vi "Read Binary Config.vi"(4 "Class Name is Included":bool, 6 "byte order (0:big-endian, network order)":T1(ring), 8 "error in (no error)":errorcluster, 10 "Binary":string, 11 "AbsComp_One Term_STR in":refnum<class "AbsComp_One Term_STR.lvclass">) -> (0 "error out":errorcluster, 2 "Remaining":string, 3 "AbsComp_One Term_STR out":refnum<class "AbsComp_One Term_STR.lvclass">)   [LabVIEW 2021, in "AbsComp_One Term_STR.lvclass"]
uses:
  AbsComp_One Term_STR.lvclass
  Abs_Types/Boolean/Abs_Boolean.lvclass
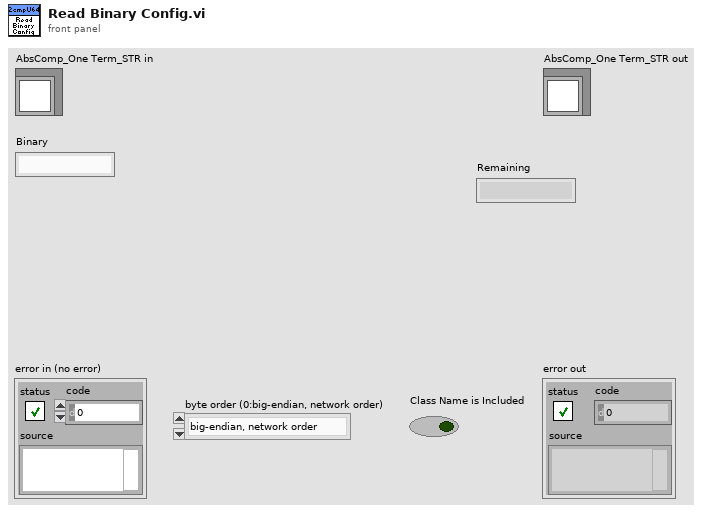
[diagram p1: front panel]
types:
  T1 = enum16{"big-endian, network order", "native, host order", "little-endian"}
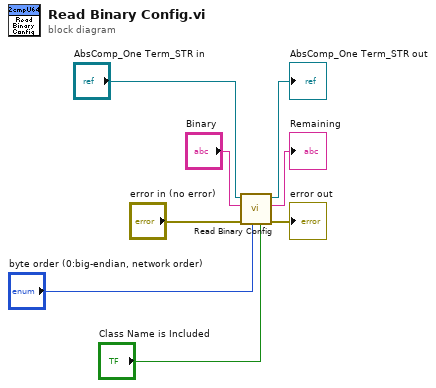
[diagram p0: block diagram]
diagram:
  n1 = call-parent "Read Binary Config.vi"("Class Name is Included"="Class Name is Included", "byte order (0:big-endian, network order)"="byte order (0:big-endian, network order)", "error in (no error)"="error in (no error)", "Binary"="Binary", "Abs_Type in"="AbsComp_One Term_STR in") -> ("error out"=→"error out":errorcluster, "Remaining"=→"Remaining":string, "Abs_Type out"=→"AbsComp_One Term_STR out":refnum<class "AbsComp_One Term_STR.lvclass">)  [unwired: 4 in]
